vi "Bead tracking mode to number of beads.vi"(1 "Bead Tracking Mode":T1) -> (0 "Number of beads":i32)   [LabVIEW 2011]
uses:
  Bead Tracking Mode.ctl
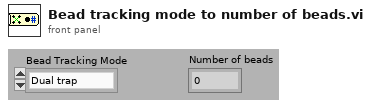
[diagram p1: front panel]
types:
  T1 = typedef "Bead Tracking Mode.ctl" = enum16{"Dual trap", "Q-trap =", "Q-trap ||", "Q-trap X", "Q-trap +", "Dual trap oO", "Single trap", "None"}
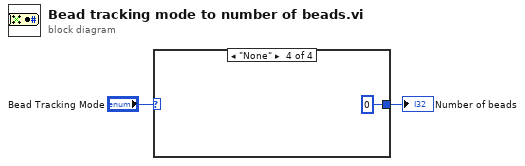
[diagram p0: block diagram]
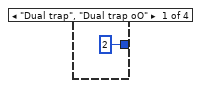
[diagram p2: hidden frame]
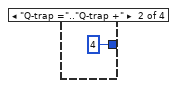
[diagram p3: hidden frame]
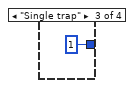
[diagram p4: hidden frame]
diagram:
  n1 = case shown="\"None\"" "Bead Tracking Mode" {
    tunnel: [2 4 1 0] -> w1
    frame "Dual trap", "Dual trap oO" {
    }
    frame "Q-trap =".."Q-trap +" {
    }
    frame "Single trap" {
    }
    frame "None" {
    }
  }
  "Number of beads" <- w1
